vi "To Waveform.vi"(8 "error in (no error)":errorcluster, 11 "Request Data in":refnum<class "DMM Measurement Data.lvclass">) -> (0 "error out":errorcluster, 1 "Success?":bool, 3 "Waveform Array":waveform(dbl)[](array[waveform]))   [LabVIEW 2020, in "DMM Msg.lvlib" / "DMM Measurement Data.lvclass"]
doc: "Interpret 'Data' as a Waveform Array. If impossible 'Success?' is set to FALSE\n\nThis implementation adds the average measurement to all Y elements from the parent implementation."
uses:
  DMM Measurement Data.lvclass
  DMM Measurement Data.lvclass/DMM Measurement Data.ctl
  PPL/HDH.Actor Framework.Core.Instrument Handler.lvlibp/Data/Instrument Data/Instrument Data.lvclass
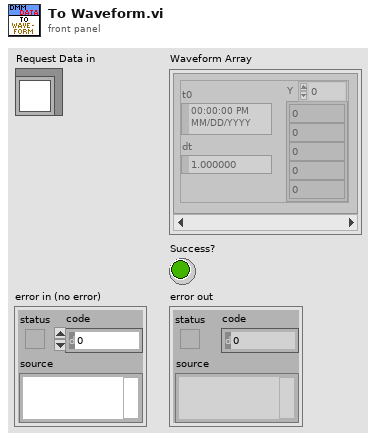
[diagram p1: front panel]
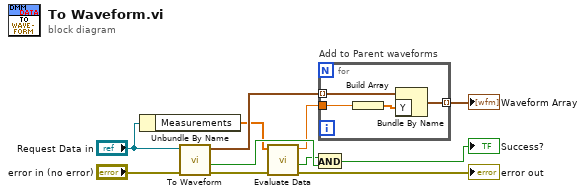
[diagram p0: block diagram]
diagram:
  n1 = Unbundle By Name("Request Data in") -> ("Measurements"=w5:dbl[])
  n2 = call-parent "To Waveform.vi"("error in (no error)"="error in (no error)", "Request Data in"="Request Data in") -> ("error out"=w2:errorcluster, "Success?"=w11:bool, "Waveform Array"=w8:waveform(dbl)[])  [unwired: 7 in]
  n3 = call "Evaluate Data.vi"("error in (no error)"=w2, "Measurements"=w5) -> ("error out"=→"error out":errorcluster, "Valid Data?"=w3:bool, "Average"=w6:dbl)  [unwired: 6 in, 1 out]
  n4 = And(x=w3, y=w11) -> (x .and. y?=→"Success?":bool)
  n5 = for "Add to Parent waveforms" {
    tunnel: w8 -> [w15] mode=indexing
    tunnel: [w14] -> w7 mode=indexing
    tunnel: w6 -> [w13]
    n6 = Build Array(w13) -> (w12:dbl[])
    n7 = Bundle By Name(cluster=w15, "Y"=w12) -> (w14:waveform(dbl))
  }
  "Waveform Array" <- w7
